vi "TestEthConnection.vi"(10 "Port":u16=80, 11 "IP address":string) -> (0 "error out":errorcluster, 1 "Answer OK?":bool)   [LabVIEW 2015, in "VIPM2.lvlib"]
uses:
  VIPM2.lvlib
panel:
  out "Answer to open":string="\n\r\n"
  # "Test Ethernet Connection"
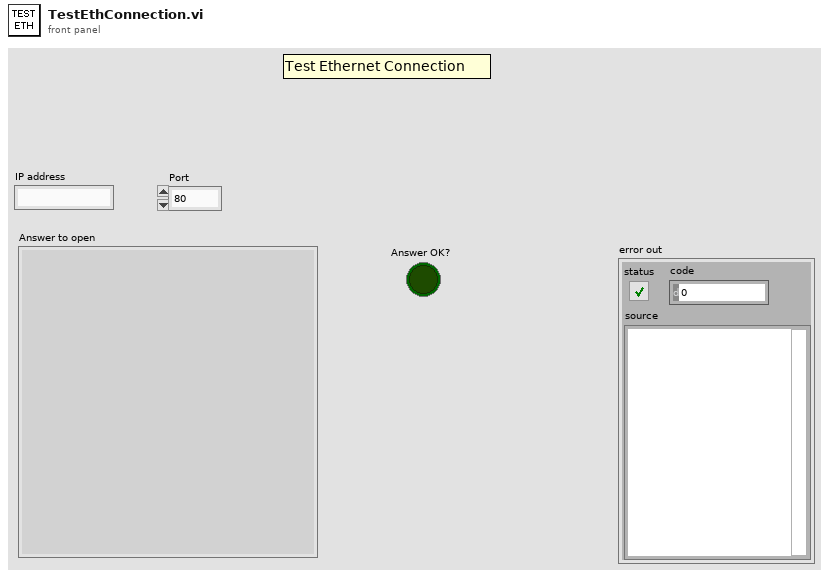
[diagram p1: front panel]
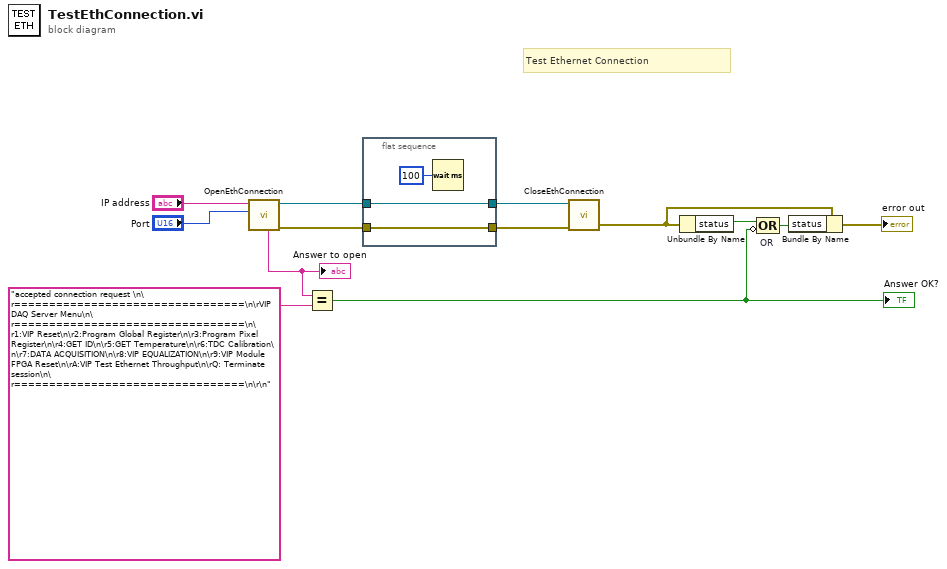
[diagram p0: block diagram]
diagram:
  # "Test Ethernet Connection"
  n1 = call "OpenEthConnection.vi"("Port"="Port", "IP address"="IP address") -> ("error out"=w5:errorcluster, "connection ID out"=w2:refnum<k5>, "Answer"=w6:string)  [unwired: 7 in]
  "Answer to open" <- w6
  n2 = Equal?(x=w6, y="accepted connection request \n\r=================================\n\rVIP DAQ Server Menu\n\r=================================\n\r1:VIP Reset\n\r2:Program Global Register\n\r3:Program Pixel Register\n\r4:GET ID\n\r5:GET Temperature\n\r6:TDC Calibration\n\r7:DATA ACQUISITION\n\r8:VIP EQUALIZATION\n\r9:VIP Module FPGA Reset\n\rA:VIP Test Ethernet Throughput\n\rQ: Terminate session\n\r=================================\n\r\n") -> (x = y?=w1:bool)
  "Answer OK?" <- w1
  n3 = flat-sequence {
    tunnel: w5 -> [w16]
    tunnel: [w16] -> w4
    tunnel: [w15] -> w3
    tunnel: w2 -> [w15]
    frame #0 {
      n4 = Wait (ms)(milliseconds to wait=u32 100) -> ()  [unwired: 1 out]
    }
  }
  n5 = call "CloseEthConnection.vi"("error in (no error)"=w4, "connection ID"=w3) -> ("error out"=w10:errorcluster)  [unwired: 9 in]
  n6 = Unbundle By Name(w10) -> ("status"=w8:bool)
  n7 = Compound Arithmetic op=OR "OR"(w8, invert w1) -> (w9:bool)
  n8 = Bundle By Name(cluster=w10, "status"=w9) -> (→"error out":errorcluster)
